vi "Run WordSearch.vi"(8 "error in (no error)":errorcluster, 11 "Solver VI":T1) -> (0 "error out":errorcluster, 2 "Completed":bool, 3 "Run Time":dbl)   [LabVIEW 2024, in "Wordle Scorer.lvlib"]
uses:
  Wordle Scorer.lvlib
  Solver VI Ref Type.ctl
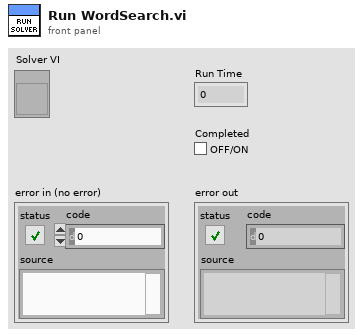
[diagram p1: front panel]
types:
  T1 = typedef "Wordle Scorer.lvlib/Solver VI Ref Type.ctl" = refnum<vi>
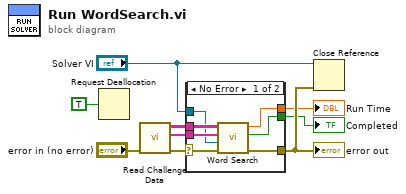
[diagram p0: block diagram]
diagram:
  n1 = Request Deallocation(TRUE ("flag")) -> ()
  n2 = call "Read Challenge Data.vi"("error in (no error)"="error in (no error)") -> ("error out"=w5:errorcluster, "Word List"=w6:string[], "Grid"=w7:string[][])  [unwired: 8 in]
  n3 = case shown="No Error" w5 {
    selector: w5 -> [w11 w17]
    tunnel: w7 -> [w16 _]
    tunnel: w6 -> [w15 _]
    tunnel: "Solver VI" -> [w14 _]
    tunnel: [w10 w17] -> w9
    tunnel: [w13 _] -> w4
    tunnel: [w12 _] -> w3
    frame No Error {
      n4 = call "Word Search.vi"("error in (no error)"=w11, "Solver VI"=w14, "Word List"=w15, "Word Search Grid"=w16) -> ("error out"=w10:errorcluster, "All Words Found"=w12:bool, "Execution Time"=w13:dbl)  [unwired: 5 in]
    }
    frame Error {
    }
  }
  "error out" <- w9
  "Run Time" <- w4
  "Completed" <- w3
  n5 = Close Reference(reference="Solver VI", error in (no error)=w9) -> ()  [unwired: 1 out]
